vi "removeEmptyElements.vi"(8 "error in (no error)":errorcluster, 10 "data":T1(array[cluster])=[[{"time"=0.0, "Channel"=refnum, "data"=0.8}, {"time"=29.998, "Channel"=refnum, "data"=0.0}], [{"time"=0.0, "Channel"=refnum, "data"=0.74}, {"time"=29.998, "Channel"=refnum, "data"=0.0}], [{"time"=29.998, "Channel"=refnum, "data"=0.8}, {"time"=33.5, "Channel"=refnum, "data"=0.0}]], 11 "DeviceData in":refnum<class "DeviceData.lvclass">) -> (0 "error out":errorcluster, 2 "data out":T1(array[cluster]), 3 "DeviceData out":refnum<class "DeviceData.lvclass">)   [LabVIEW 2009, in "DataMappers.lvlib" / "DeviceData.lvclass"]
uses:
  DeviceData.lvclass
  DatabaseHelpers/Database Objects/Channel/Channel.lvclass
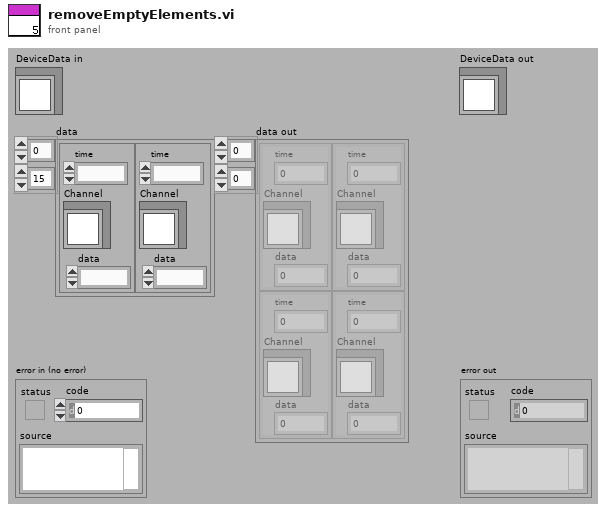
[diagram p1: front panel]
types:
  T1 = cluster{"time":dbl, "Channel":refnum<class "Channel.lvclass">, "data":dbl}[][]
  T2 = cluster{"time":dbl, "Channel":refnum<class "Channel.lvclass">, "data":dbl}
  T3 = cluster{"time":dbl, "Channel":refnum<class "Channel.lvclass">, "data":dbl}[]
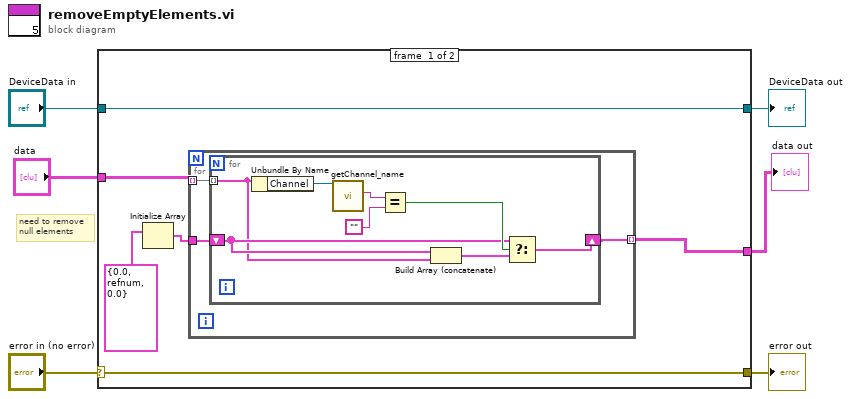
[diagram p0: block diagram]
diagram:
  # "need to remove\nnull elements"
  n1 = case shown="No Error" "error in (no error)" {
    selector: "error in (no error)" -> [w11 w25]
    tunnel: [w11 w25] -> w5
    tunnel: [w12 w24] -> w3
    tunnel: "DeviceData in" -> [w12 w24]
    tunnel: "data" -> [w10 _]
    tunnel: [w7 _] -> w1
    frame #0 {
      n2 = Initialize Array(T2 {"time"=0.0, "Channel"=refnum, "data"=0.0}) -> (w8:T3)  [unwired: 1 in]
      n3 = for {
        tunnel: w10 -> [w15] mode=indexing
        tunnel: w8 -> [w14]
        tunnel: [w13] -> w7 mode=indexing
        n4 = for {
          tunnel: w15 -> [w16] mode=indexing
          shift-right: [w19] -> w13
          shift-left: w14 -> [w17]
          n5 = Unbundle By Name(w16) -> ("Channel"=w23:refnum<class "Channel.lvclass">)
          n6 = call "getChannel_name.vi"("Channel.lvclass in"=w23) -> ("channel_name"=w21:string)  [unwired: 8 in, 2 out]
          n7 = Equal?(x=w21, y="") -> (x = y?=w20:bool)
          n8 = Build Array (concatenate)(w17, w16) -> (w18:T3)
          n9 = Select(t=w17, s=w20, f=w18) -> (s? t:f=w19:T3)
        }
      }
    }
    frame #1 {
    }
  }
  "error out" <- w5
  "DeviceData out" <- w3
  "data out" <- w1
